vi "Build Channel Settings.vi"(8 "error in":errorcluster, 10 "Channel Settings":T1) -> (0 "error out":errorcluster, 2 "Channel Settings Table":string[][](array[string]))   [LabVIEW 2026]
uses:
  Types/ChannelSettings.ctl
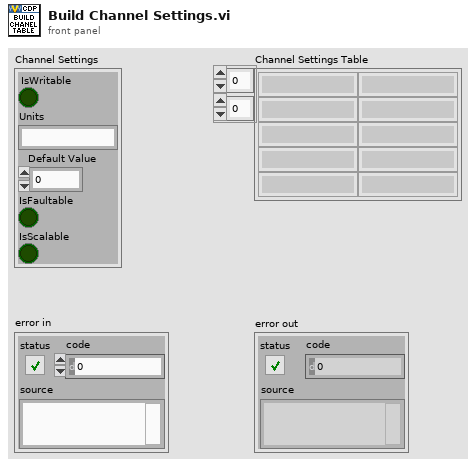
[diagram p1: front panel]
types:
  T1 = typedef "ChannelSettings.ctl" = cluster{"IsWritable":bool, "Units":string, "Default Value":dbl, "IsFaultable":bool, "IsScalable":bool}
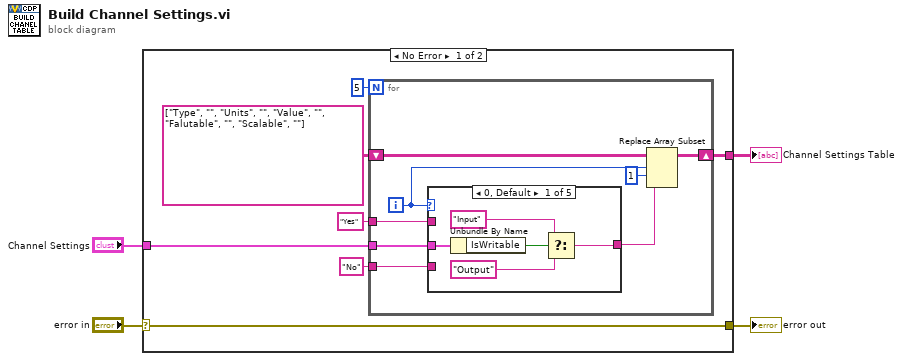
[diagram p0: block diagram]
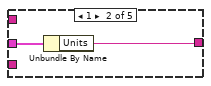
[diagram p2: hidden frame]
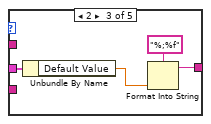
[diagram p3: hidden frame]
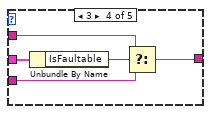
[diagram p4: hidden frame]
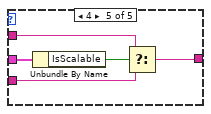
[diagram p5: hidden frame]
diagram:
  n1 = case shown="No Error" "error in" {
    selector: "error in" -> [w5 w41]
    tunnel: "Channel Settings" -> [w11 _]
    tunnel: [w6 _] -> w3
    tunnel: [w5 w41] -> w1
    frame No Error {
      n2 = for {
        N: 5 -> [_]
        tunnel: w11 -> [w19]
        shift-right: [w17] -> w6
        shift-left: string[][] [["Type", ""], ["Units", ""], ["Value", ""], ["Falutable", ""], ["Scalable", ""]] -> [w18]
        tunnel: "Yes" -> [w16]
        tunnel: "No" -> [w15]
        i -> [w13]
        n3 = case shown="0, Default" w13 {
          tunnel: w19 -> [w24 w26 w30 w35 w40]
          tunnel: w16 -> [_ _ _ w32 w37]
          tunnel: w15 -> [_ _ _ w33 w38]
          tunnel: [w22 w25 w27 w31 w36] -> w14
          frame 0, Default {
            n4 = Unbundle By Name(w24) -> ("IsWritable"=w23:bool)
            n5 = Select(t="Input", s=w23, f="Output") -> (s? t:f=w22:string)
          }
          frame 1 {
            n6 = Unbundle By Name(w26) -> ("Units"=w25:string)
          }
          frame 2 {
            n7 = Unbundle By Name(w30) -> ("Default Value"=w28:dbl)
            n8 = Format Into String(format string="%;%f", w28) -> (resulting string=w27:string)  [unwired: 2 in, 1 out]
          }
          frame 3 {
            n9 = Unbundle By Name(w35) -> ("IsFaultable"=w34:bool)
            n10 = Select(t=w32, s=w34, f=w33) -> (s? t:f=w31:string)
          }
          frame 4 {
            n11 = Unbundle By Name(w40) -> ("IsScalable"=w39:bool)
            n12 = Select(t=w37, s=w39, f=w38) -> (s? t:f=w36:string)
          }
        }
        n13 = Replace Array Subset(array=w18, new element=w14, index (row)=w13, index (col)=1 ("disabled index (col)")) -> (w17:string[][])
      }
    }
    frame Error {
    }
  }
  "Channel Settings Table" <- w3
  "error out" <- w1
